vi "initialize.vi"(0 "MySociety":refnum<class "HB_Society.lvclass">, 3 "initializationData":variant, 5 "error in (no error)":errorcluster, 7 "binaryString":string, 8 "I8 Array":i8[](array[numeric]), 9 "prependSize? (T)":bool, 11 "byteOrder (0:big-endian, network order)":T1(ring)) -> (14 "dup MySociety":refnum<class "HB_Society.lvclass">, 17 "found?":bool, 19 "error out":errorcluster)   [LabVIEW 2009, in "HB_BaseClass_Examples.lvlib" / "HB_Society.lvclass"]
doc: "This is a dynamic dispatch VI to be implemented by child classes to initialize their attributes.\n\n<B>Recommendation:</B> Use Variant for initialization data."
uses:
  HB_Society.lvclass
  lib.lib/HGF_LVC/HGF_BaseClasses/HGF_Composite/HGF_Composite.lvclass
  HB_Society.lvclass/HB_Society.ctl
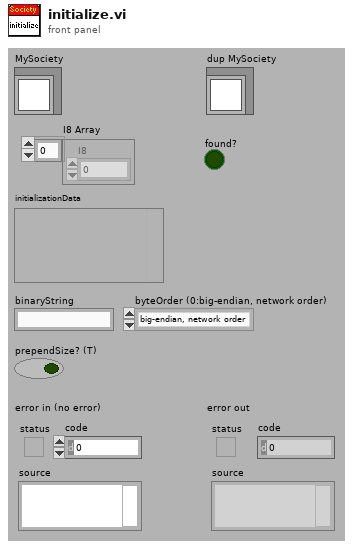
[diagram p1: front panel]
types:
  T1 = enum16{"big-endian, network order", "native, host order", "little-endian"}
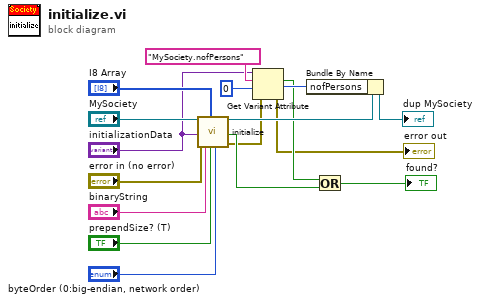
[diagram p0: block diagram]
diagram:
  n1 = call-parent "initialize.vi"("HGF_Base"="MySociety", "initializationData"="initializationData", "error in (no error)"="error in (no error)", "binaryString"="binaryString", "I8 Array"="I8 Array", "prependSize? (T)"="prependSize? (T)", "byteOrder (0:big-endian, network order)"="byteOrder (0:big-endian, network order)") -> ("dup HGF_Base"=w10:refnum<class "HB_Society.lvclass">, "found?"=w7:bool, "error out"=w6:errorcluster)  [unwired: 1 in, 9 out]
  n2 = Get Variant Attribute(Variant="initializationData", name="MySociety.nofPersons", default value (empty Variant)=0, error in=w6) -> (found=w8:bool, value=w14:i32, error out=→"error out":errorcluster)  [unwired: 1 out]
  n3 = Bundle By Name(cluster=w10, "nofPersons"=w14) -> (→"dup MySociety":refnum<class "HB_Society.lvclass">)
  n4 = Or(x=w8, y=w7) -> (x .or. y?=→"found?":bool)
